vi "Get AccessSDO.vi"(8 "error in":errorcluster, 11 "OD Entry in":refnum<class "OD Entry.lvclass">) -> (0 "error out":errorcluster, 2 "Access SDO":T1, 3 "OD Entry out":refnum<class "OD Entry.lvclass">)   [LabVIEW 2024, in "Electronic Datasheet.lvlib" / "OD Entry.lvclass"]
uses:
  OD Entry.lvclass
  OD Entry.lvclass/OD Entry.ctl
  Access SDO.ctl
  Electronic Datasheet.lvlib
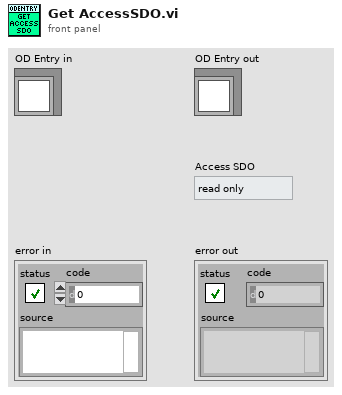
[diagram p1: front panel]
types:
  T1 = typedef "Electronic Datasheet.lvlib/Access SDO.ctl" = enum16{"read only", "write only", "read/write", "read/write on process input", "read/write on process output", "constant value", "no", "UNKNOWN"}
  T2 = enum16{"read only", "write only", "read/write", "read/write on process input", "read/write on process output", "constant value", "no", "UNKNOWN"}
  T3 = enum16{"ro", "wo", "rw", "rwr", "rww", "const", "UNKNOWN"}
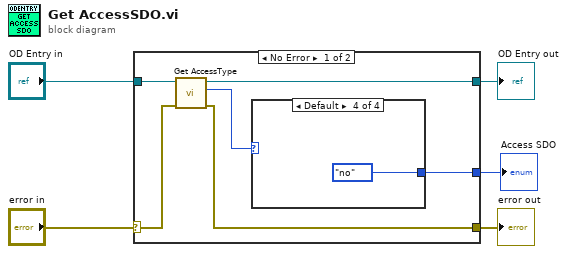
[diagram p0: block diagram]
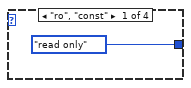
[diagram p2: hidden frame]
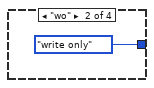
[diagram p3: hidden frame]
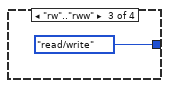
[diagram p4: hidden frame]
diagram:
  n1 = case shown="No Error" "error in" {
    selector: "error in" -> [w10 w17]
    tunnel: [w6 w17] -> w4
    tunnel: [w7 w16] -> w2
    tunnel: "OD Entry in" -> [w11 w16]
    tunnel: [w8 _] -> w1
    frame No Error {
      n2 = call "Get AccessType.vi"("Error In"=w10, "reference in"=w11) -> ("Error Out"=w6:errorcluster, "AccessType"=w9:T3, "reference out"=w7:refnum<class "OD Entry.lvclass">)  [unwired: 7 in]
      n3 = case shown="Default" w9 {
        tunnel: [T2."read only" ("Access SDO") Access_SDO."write only" ("Access SDO") Access_SDO."read/write" ("Access SDO") Access_SDO."no" ("Access SDO")] -> w8
        frame "ro", "const" {
        }
        frame "wo" {
        }
        frame "rw".."rww" {
        }
        frame Default {
        }
      }
    }
    frame Error {
    }
  }
  "error out" <- w4
  "OD Entry out" <- w2
  "Access SDO" <- w1
